vi "test_ccd_acquireSpectrum.vi"(8 "error in":errorcluster, 11 "CCD in":refnum<class "CCD.lvclass">) -> (0 "error out":errorcluster, 3 "CCD out":refnum<class "CCD.lvclass">)   [LabVIEW 2023, in "horiba.test.lvlib"]
uses:
  horiba.test.lvlib
  Classes/CCD/CCD.lvclass
  Classes/CCD/acquisitionData.ctl
  Classes/CCD/CCDImageData.ctl
  f7563d15-716f-4b44-beb1-7a38c7aa8869.vi
  <vilib>/addons/_JKI Toolkits/Caraya/classes/Test/Test.lvclass
  <vilib>/addons/_JKI Toolkits/Caraya/classes/Assert/Assert.lvclass
  <userlib>/_OpenG.lib/lvdata/lvdata.llb/openg_variant.lvlib
panel:
  out "Aquisitions":T1[](array[typedef])
  # "Connector Pane"
  # "Locals"
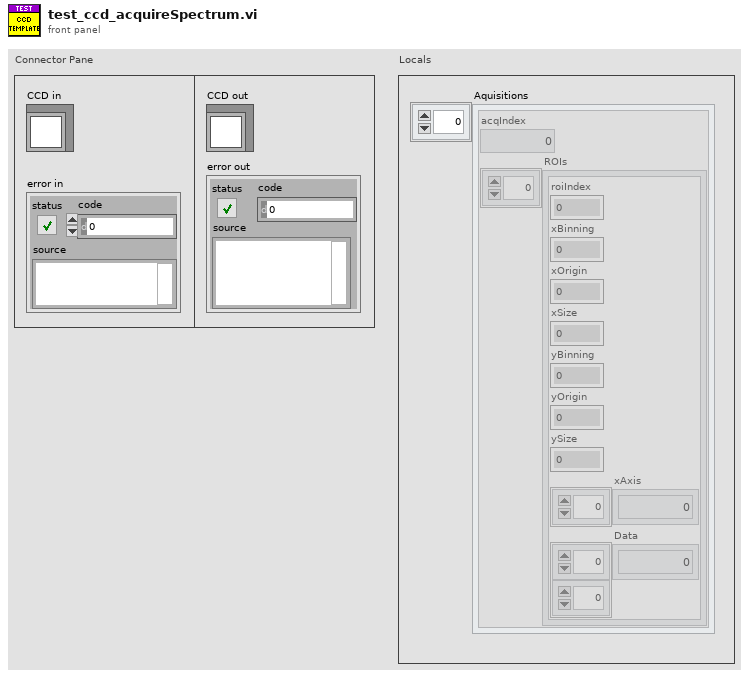
[diagram p1: front panel]
types:
  T1 = typedef "horiba.lvlib/CCD.lvclass/acquisitionData.ctl" = cluster{"acqIndex":i32, "ROIs":T2[]}
  T2 = typedef "horiba.lvlib/CCD.lvclass/CCDImageData.ctl" = cluster{"roiIndex":i32, "xBinning":i32, "xOrigin":i32, "xSize":i32, "yBinning":i32, "yOrigin":i32, "ySize":i32, "xAxis":dbl[], "Data":dbl[][]}
  T3 = cluster{"ROI-index":i32, "xOrigin":i32, "yOrigin":i32, "xSize":i32, "ySize":i32, "xBin":i32, "yBin":i32}
  T4 = typedef "acquisitionData.ctl" = cluster{"acqIndex":i32, "ROIs":T2[]}
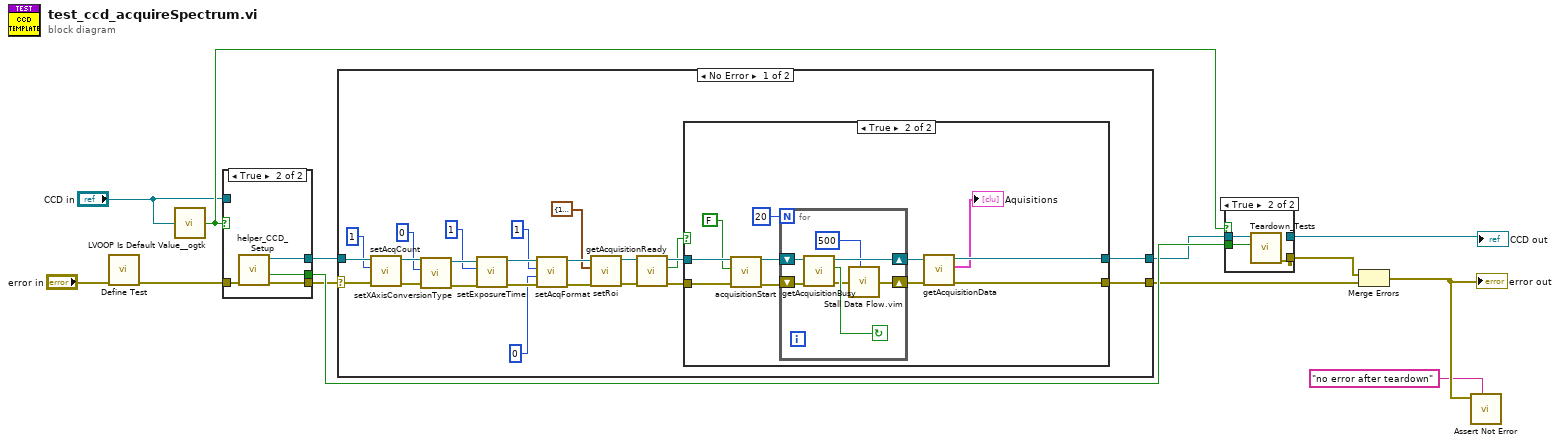
[diagram p0: block diagram]
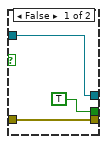
[diagram p2: hidden frame]
diagram:
  n1 = call <vilib>:"Define Test.vi"("error in (no error)"="error in") -> ("error out"=w8:errorcluster)  [unwired: 9 in, 1 out]
  n2 = call <userlib>:"LVOOP Is Default Value__ogtk.vi"("Object"="CCD in") -> ("Is Default Value?"=w9:bool)
  n3 = case shown="True" w9 {
    tunnel: w8 -> [w15 w20]
    tunnel: [w15 w19] -> w4
    tunnel: [w16 w18] -> w6
    tunnel: [TRUE ("Module Was Already Running?") w17] -> w10
    tunnel: "CCD in" -> [w16 _]
    frame False {
    }
    frame True {
      n4 = call "helper_CCD_Setup.vi"("error in"=w20) -> ("error out"=w19:errorcluster, "Module Was Already Running?"=w17:bool, "CCD out"=w18:refnum<class "CCD.lvclass">)  [unwired: 7 in, 1 out]
    }
  }
  n5 = case shown="No Error" w4 {
    selector: w4 -> [w43 w65]
    tunnel: [w22 w64] -> w5
    tunnel: w6 -> [w42 w64]
    tunnel: [w23 w65] -> w3
    frame No Error {
      n6 = call "setAcqCount.vi"("error in (no error)"=w43, "count"=1, "CCD in"=w42) -> ("error out"=w40:errorcluster, "CCD out"=w39:refnum<class "CCD.lvclass">)  [unwired: 5 in, 2 out]
      n7 = call "setXAxisConversionType.vi"("error in (no error)"=w40, "type"=0, "CCD in"=w39) -> ("error out"=w37:errorcluster, "CCD out"=w36:refnum<class "CCD.lvclass">)  [unwired: 5 in, 2 out]
      n8 = call "setExposureTime.vi"("error in (no error)"=w37, "exposure time [ms] or [us]"=1, "CCD in"=w36) -> ("error out"=w34:errorcluster, "CCD out"=w33:refnum<class "CCD.lvclass">)  [unwired: 5 in, 2 out]
      n9 = call "setAcqFormat.vi"("error in (no error)"=w34, "format"=0, "number of ROIs"=1, "CCD in"=w33) -> ("error out"=w30:errorcluster, "CCD out"=w29:refnum<class "CCD.lvclass">)  [unwired: 4 in, 2 out]
      n10 = call "setRoi.vi"("error in (no error)"=w30, "roiConfig"=T3 {"ROI-index"=1, "xOrigin"=0, "yOrigin"=0, "xSize"=1024, "ySize"=256, "xBin"=1, "yBin"=256}, "CCD in"=w29) -> ("error out"=w27:errorcluster, "CCD out"=w26:refnum<class "CCD.lvclass">)  [unwired: 5 in, 2 out]
      n11 = call "getAcquisitionReady.vi"("error in (no error)"=w27, "CCD in"=w26) -> ("error out"=w25:errorcluster, "ready"=w21:bool, "CCD out"=w24:refnum<class "CCD.lvclass">)  [unwired: 7 in]
      n12 = case shown="True" w21 {
        tunnel: w25 -> [w44 w56]
        tunnel: w24 -> [w45 w55]
        tunnel: [w44 w49] -> w23
        tunnel: [w45 w47] -> w22
        frame False {
        }
        frame True {
          n13 = call "acquisitionStart.vi"("error in (no error)"=w56, "openShutter"=FALSE, "CCD in"=w55) -> ("error out"=w51:errorcluster, "CCD out"=w50:refnum<class "CCD.lvclass">)  [unwired: 5 in, 2 out]
          n14 = for {
            N: 20 -> [_]
            shift-right: [w59] -> w52
            shift-left: w51 -> [w62]
            shift-right: [w58] -> w48
            shift-left: w50 -> [w63]
            stop <- w61 continue-if-true
            n15 = call "getAcquisitionBusy.vi"("error in (no error)"=w62, "CCD in"=w63) -> ("error out"=w60:errorcluster, "isBusy"=w61:bool, "CCD out"=w58:refnum<class "CCD.lvclass">)  [unwired: 7 in]
            n16 = call "Stall Data Flow.vim"("value in"=w60, "milliseconds to wait"=u32 500) -> ("value out"=w59:errorcluster)  [unwired: 1 out]
          }
          n17 = call "getAcquisitionData.vi"("error in (no error)"=w52, "CCD in"=w48) -> ("error out"=w49:errorcluster, "Aquisitions"=→"Aquisitions":T4[], "CCD out"=w47:refnum<class "CCD.lvclass">)  [unwired: 6 in, 1 out]
        }
      }
    }
    frame Error {
    }
  }
  n18 = case shown="True" w9 {
    tunnel: w5 -> [w66 w69]
    tunnel: [_ w68] -> w7
    tunnel: w10 -> [_ w67]
    tunnel: [w66 _] -> w1
    frame False {
    }
    frame True {
      n19 = call "Teardown_Tests.vi"("Module Was Already Running?"=w67, "horiba.lvlib:GenericDevice"=w69) -> ("error out"=w68:errorcluster)  [unwired: 8 in, 1 out]
    }
  }
  "CCD out" <- w1
  n20 = Merge Errors(w7, w3) -> (w12:errorcluster)
  "error out" <- w12
  n21 = call <vilib>:"Assert Not Error.vi"("Label"="no error after teardown", "Not Error?"=w12) -> ()  [unwired: 8 in, 2 out]
